vi "form_filename.vi"(3 "Parameters to Change":T1={"PB parameter to change"=0, "Column of\nData to Change"=0, "Column of\nDelay to Change"=9, "6713 DAC Ch\nto Change"=7, "column for Wvfrm\n(red mot cooling)"=10, "# of PB arrays"=1, "column for Wvrm\nODT"=10, "TrimCurrent\nCh to Chng"=1} {"TrimCurrent\nCh to Chng" min=1 max=2; "PB parameter to change" min=0 max=4}, 4 "iteration #":i32, 5 "6713 DAC Array":dbl[](array[numeric]), 6 "Current PulseBlaster Array":T2(array[cluster]), 7 "Base File Name":string="redMOTtemp0441" caption="Base File Name (filename, base delay of column 10, and .dat will be added as extension.") -> (0 "filename component":string, 1 "6713 DAC CH0":string, 2 "FrontPanelName":string)   [LabVIEW 2013]
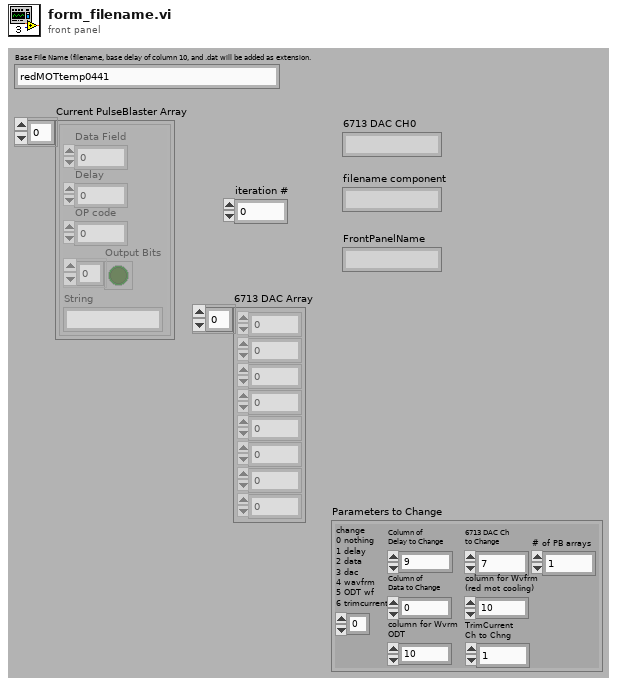
[diagram p1: front panel]
types:
  T1 = cluster{"PB parameter to change":i8, "Column of\nData to Change":i32, "Column of\nDelay to Change":i32, "6713 DAC Ch\nto Change":i32, "column for Wvfrm\n(red mot cooling)":i32, "# of PB arrays":i32, "column for Wvrm\nODT":i32, "TrimCurrent\nCh to Chng":i32}
  T2 = cluster{"Data Field":u32, "Delay":dbl, "OP code":u8, "Output Bits":bool[], "String":string}[]
  T3 = cluster{"Data Field":u32, "Delay":dbl, "OP code":u8, "Output Bits":bool[], "String":string}
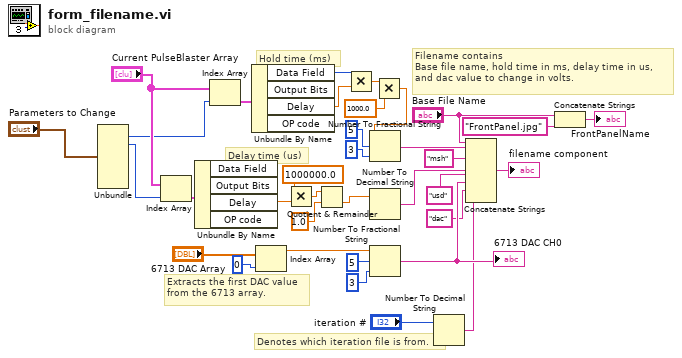
[diagram p0: block diagram]
diagram:
  # "Delay time (us)"
  # "Hold time (ms)"
  # "Filename contains\nBase file name, hold time in ms, delay time in us,\nand dac value to change in volts."
  # "Extracts the first DAC value\nfrom the 6713 array."
  # "Denotes which iteration file is from."
  n1 = Unbundle("Parameters to Change") -> ("Column of\nData to Change"=w6:i32, "Column of\nDelay to Change"=w5:i32)  [unwired: 6 out]
  n2 = Index Array(array="Current PulseBlaster Array", index=w5) -> (element=w26:T3)
  n3 = Unbundle By Name(w26) -> ("Delay"=w27:dbl)  [unwired: 3 out]
  n4 = Index Array(array="Current PulseBlaster Array", index=w6) -> (element=w19:T3)
  n5 = Unbundle By Name(w19) -> ("Data Field"=w23:u32, "Delay"=w24:dbl)  [unwired: 2 out]
  n6 = Index Array(array="6713 DAC Array", index=0 ("Index")) -> (element=w18:dbl)
  n7 = Multiply(x=1000000.0, y=w27) -> (x*y=w30:dbl)
  n8 = Quotient & Remainder(x=w30, y=1.0) -> (floor(x/y)=w31:dbl)  [unwired: 1 out]
  n9 = Multiply(x=w23, y=w24) -> (x*y=w32:dbl)
  n10 = Number To Decimal String(number=w31) -> (decimal integer string=w13:string)  [unwired: 1 in]
  n11 = Number To Fractional String(number=w18, width (-)=i16 5, precision (6)=i16 3) -> (F-format string=w20:string)  [unwired: 1 in]
  "6713 DAC CH0" <- w20
  n12 = Multiply(x=w32, y=1000.0) -> (x*y=w33:dbl)
  n13 = Number To Fractional String(number=w33, width (-)=i16 5, precision (6)=i16 3) -> (F-format string=w10:string)  [unwired: 1 in]
  n14 = Number To Decimal String(number="iteration #") -> (decimal integer string=w16:string)  [unwired: 1 in]
  n15 = Concatenate Strings("Base File Name", w10, "msh" ("Substring"), w13, "usd" ("Substring"), w20, "dac" ("Substring"), w16) -> (→"filename component":string)
  n16 = Concatenate Strings("Base File Name", "FrontPanel.jpg" ("string")) -> (→"FrontPanelName":string)
